vi "Read Generation State.vi"(8 "error in (no error)":errorcluster, 11 "SV Signal in":refnum<class "SV Signal.lvclass">) -> (0 "error out":errorcluster, 2 "generation state":T1=enum."Pre-Measurement Settling", 3 "SV Signal out":refnum<class "SV Signal.lvclass">)   [LabVIEW 2017, in "SV Signal.lvclass"]
uses:
  <vilib>/addons/_NISVFA/_Generation/Signal Generation/SV Signal/SV Signal.lvclass
  <vilib>/addons/_NISVFA/_Generation/Signal Generation/SV Signal/sv_Generation State.ctl
  <vilib>/addons/_NISVFA/_Generation/Signal Generation/SV Signal/SV Signal.lvclass/SV Signal.ctl
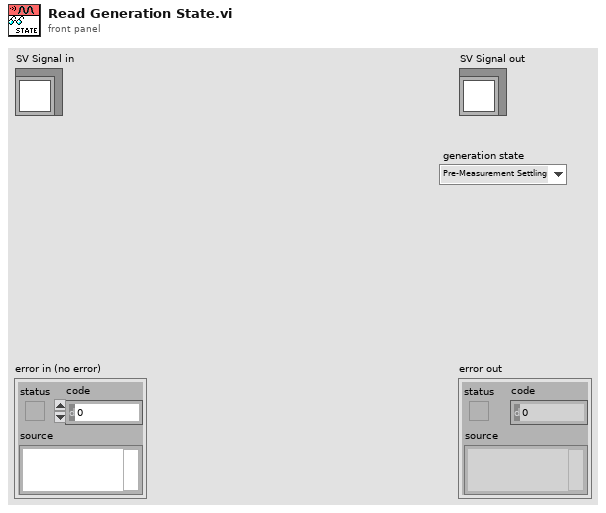
[diagram p1: front panel]
types:
  T1 = typedef "SV Signal.lvclass/sv_Generation State.ctl" = enum16{"Idle", "Ramp Up", "Pre-Measurement Settling", "Measurement", "Post-Measurement Settling", "Discrete Sweep Transition", "Ramp Down", "Update"}
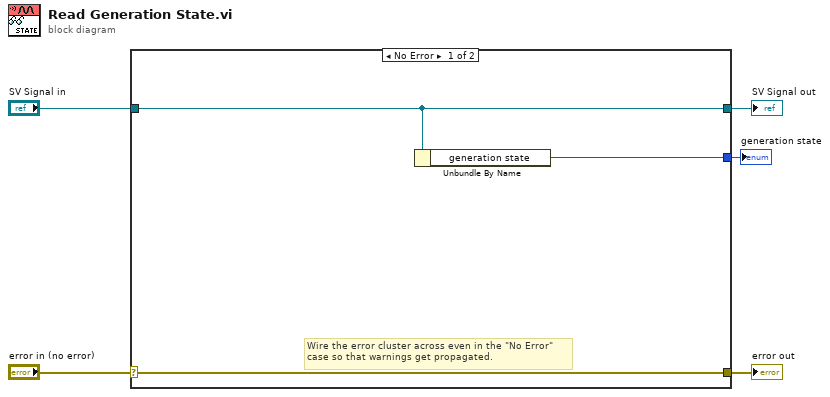
[diagram p0: block diagram]
diagram:
  n1 = case shown="No Error" "error in (no error)" {
    selector: "error in (no error)" -> [w8 w10]
    tunnel: [w8 w10] -> w4
    tunnel: [w7 w9] -> w2
    tunnel: "SV Signal in" -> [w7 w9]
    tunnel: [w6 _] -> w1
    frame No Error {
      # "Wire the error cluster across even in the \"No Error\"\ncase so that warnings get propagated."
      n2 = Unbundle By Name(w7) -> ("generation state"=w6:T1)
    }
    frame Error {
    }
  }
  "error out" <- w4
  "SV Signal out" <- w2
  "generation state" <- w1
